vi "Begin.vi"() -> (0 "error out":errorcluster)   [LabVIEW 2013]
doc: "Called before other user functions, this VI is expected to open initial I/O refnums, load in file data, and do all program initialization. Notice that the <B>error out</B> terminal is simply used for data flow. Wiring it to other structures or subVIs ensures that this VI runs first."
uses:
  <vilib>/Rock Robotics/SystemInterfaces/DIO/FPGA_DIOPWMChannel.ctl
  <vilib>/Rock Robotics/WPI/DriverStation/WPI_DriverStationRobotMode2.ctl
  <vilib>/Rock Robotics/WPI/Joystick/WPI_JoystickDeviceEnum.ctl
  <vilib>/Rock Robotics/WPI/Solenoid/WPI_SolenoidChannel.ctl
  <vilib>/Rock Robotics/SystemInterfaces/DIO/FPGA_DIOChannel.ctl
  <vilib>/Rock Robotics/SystemInterfaces/DIO/FPGA_DIORelayChannel.ctl
  <vilib>/Rock Robotics/SystemInterfaces/Typedef/FPGA_TypedefAnalogModule.ctl
  <vilib>/Rock Robotics/SystemInterfaces/AI/FPGA_AIChannel.ctl
  <vilib>/Rock Robotics/WPI/RobotDrive/WPI_RobotDriveOpen2MotorWithTalon.vi
  Robot Global Data.vi
  <vilib>/Rock Robotics/WPI/MotorControl/WPI_MotorControlOpen Jaguar.vi
  <vilib>/Rock Robotics/WPI/Solenoid/WPI_SolenoidOpenDouble.vi
  <vilib>/Rock Robotics/WPI/Compressor/WPI_CompressorGetSetRefNum.vi
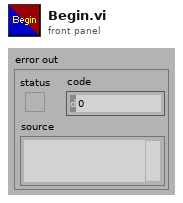
[diagram p1: front panel]
types:
  T1 = typedef "FPGA_AIChannel.ctl" = enum8{"AI 1", "AI 2", "AI 3", "AI 4", "AI 5", "AI 6", "AI 7", "AI 8", "Invalid"}
  T2 = typedef "FPGA_TypedefAnalogModule.ctl" = enum16{"Analog Module 1", "Analog Module 2"}
  T3 = typedef "FPGA_DIOChannel.ctl" = enum8{"DIO 1", "DIO 2", "DIO 3", "DIO 4", "DIO 5", "DIO 6", "DIO 7", "DIO 8", "DIO 9", "DIO 10", "DIO 11", "DIO 12", "DIO 13", "DIO 14", "Invalid"}
  T4 = typedef "WPI_SolenoidChannel.ctl" = enum8{"Solenoid 1", "Solenoid 2", "Solenoid 3", "Solenoid 4", "Solenoid 5", "Solenoid 6", "Solenoid 7", "Solenoid 8", "Invalid"}
  T5 = typedef "FPGA_DIORelayChannel.ctl" = enum8{"Relay 1", "Relay 2", "Relay 3", "Relay 4", "Relay 5", "Relay 6", "Relay 7", "Relay 8", "Invalid"}
  T6 = typedef "FPGA_DIOPWMChannel.ctl" = enum8{"PWM 1", "PWM 2", "PWM 3", "PWM 4", "PWM 5", "PWM 6", "PWM 7", "PWM 8", "PWM 9", "PWM 10", "Invalid"}
  T7 = typedef "WPI_JoystickDeviceEnum.ctl" = enum16{"USB 1", "USB 2", "USB 3", "USB 4", "Kinect 1", "Kinect 2"}
  T8 = typedef "WPI_DriverStationRobotMode2.ctl" = enum16{"Autonomous Disabled", "Autonomous Enabled", "Teleop Disabled", "Teleop Enabled", "Timeout", "Finish", "Test Disabled", "Test Enabled"}
  T9 = typedef "WPI_AnalogChannelDevRef.ctl" = cluster{"DevStatus":errorcluster, "Analog Module":T2, "Analog Channel":T1}
  T10 = typedef "WPI_DigitalInputDevRef.ctl" = cluster{"DevStatus":errorcluster, "DIO Channel":T3, "Digital Module":T11}
  T11 = typedef "FPGA_TypedefDigitalModule.ctl" = enum16{"Digital Module 1", "Digital Module 2"}
  T12 = typedef "WPI_MotorControlDeviceRef.ctl" = cluster{"DeviceStatus":errorcluster, "Type":enum16{"PWM", "CAN"}, "PWM":cluster{"Digital Module":T11, "PWM Channel":T6, "DeadBand":T13}, "CAN":cluster{"Device Number":u8, "Control Mode":T14, "Semaphore":T15, "Max Vout":dbl}, "Invert":bool, "TransformRef":T16, "InvTransformRef":T16}
  T13 = typedef "WPI_PWMDeadband.ctl" = cluster{"Name":string, "maxPositivePwm":i32, "minPositivePwm":i32, "centerPwm":i32, "maxNegativePwm":i32, "minNegativePwm":i32, "angularRange":u16}
  T14 = typedef "WPI_CANJaguar_ControlMode.ctl" = enum8{"Percent VBus", "Current", "Speed", "Position", "Voltage"}
  T15 = typedef "Semaphore RefNum" = refnum<k1>
  T16 = typedef "WPI_PWMTransform_ConPane.ctl" = refnum<vi>
  T17 = typedef "WPI_ServoDeviceRef.ctl" = cluster{"DeviceStatus":errorcluster, "Digital Module":T11, "PWM Channel":T6, "DeadBand":T13}
  T18 = typedef "WPI_RobotDriveDevRef.ctl" = cluster{"DevStatus":errorcluster, "Motors[]":T12[], "Square Inputs":bool, "Max Output":dbl, "Isochronous":bool}
  T19 = typedef "WPI_JoystickDevRef.ctl" = cluster{"Device":T7}
  T20 = typedef "WPI_RelayDevRef.ctl" = cluster{"DevStatus":errorcluster, "Relay Channel":T5, "Digital Module":T11, "Relay Direction":T21}
  T21 = typedef "WPI_RelayDirection.ctl" = enum16{"Both directions", "Forward only", "Reverse only"}
  T22 = typedef "WPI_CompressorDevRef.ctl" = cluster{"DevStatus":errorcluster, "DigitalInputDevRef":T10, "RelayDevRef":T20}
  T23 = typedef "WPI_SolenoidDevRef.ctl" = cluster{"DevStatus":errorcluster, "Solenoid Module":T24, "Forward Solenoid Channel":T4, "Reverse Solenoid Channel":T4}
  T24 = typedef "FPGA_TypedefSolenoidModule.ctl" = enum16{"Solenoid Module 1", "Solenoid Module 2"}
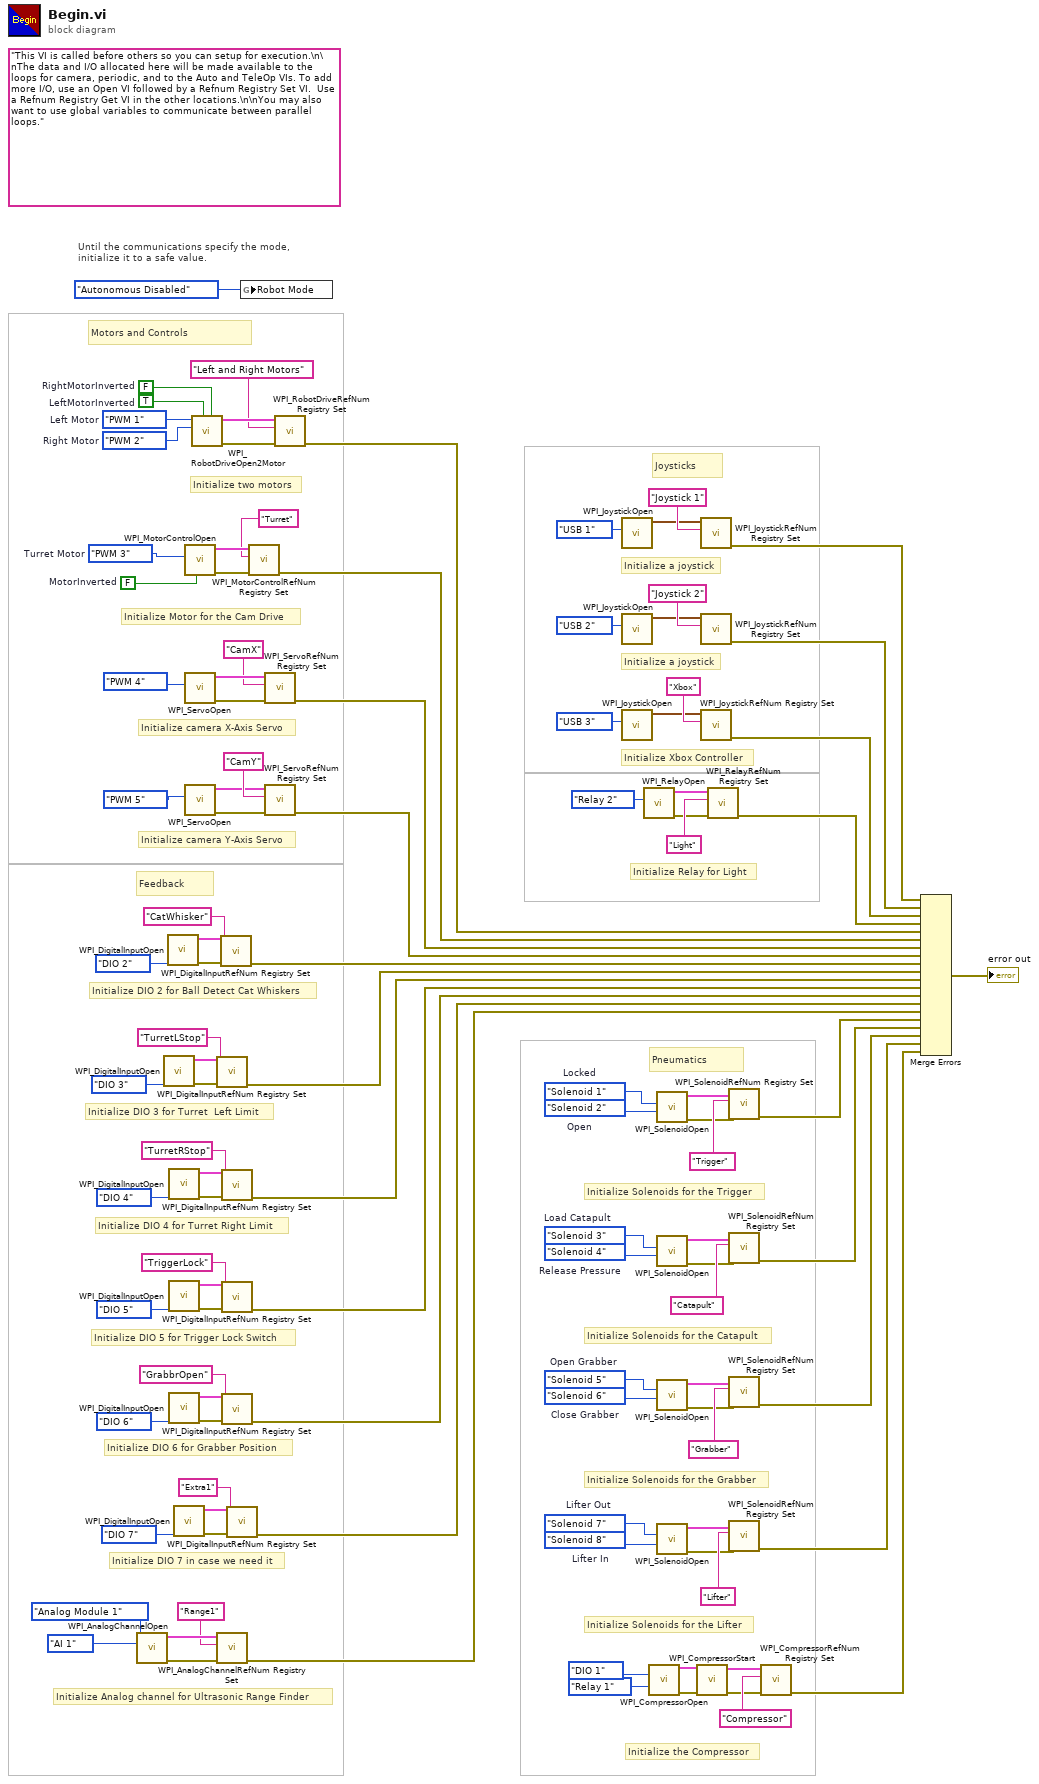
[diagram p0: block diagram]
diagram:
  w32 = WPI_SolenoidChannel."Solenoid 8"  # Lifter In
  w33 = WPI_SolenoidChannel."Solenoid 6"  # Close Grabber
  w34 = WPI_SolenoidChannel."Solenoid 4"  # Release Pressure
  w35 = WPI_SolenoidChannel."Solenoid 2"  # Open
  w51 = FALSE  # MotorInverted
  w55 = FPGA_DIOPWMChannel."PWM 3"  # Turret Motor
  w83 = WPI_SolenoidChannel."Solenoid 7"  # Lifter Out
  w86 = WPI_SolenoidChannel."Solenoid 5"  # Open Grabber
  w89 = WPI_SolenoidChannel."Solenoid 3"  # Load Catapult
  w92 = WPI_SolenoidChannel."Solenoid 1"  # Locked
  (unwired) "This VI is called before others so you can setup for execution.\n\nThe data and I/O allocated here will be made available to the loops for camera, periodic, and to the Auto and TeleOp VIs. To add more I/O, use an Open VI followed by a Refnum Registry Set VI.  Use a Refnum Registry Get VI in the other locations.\n\nYou may also want to use global variables to communicate between parallel loops."
  w105 = FPGA_DIOPWMChannel."PWM 2"  # Right Motor
  w106 = FPGA_DIOPWMChannel."PWM 1"  # Left Motor
  w110 = TRUE  # LeftMotorInverted
  w111 = FALSE  # RightMotorInverted
  # "Initialize DIO 2 for Ball Detect Cat Whiskers"
  # "Initialize the Compressor"
  # "Joysticks"
  # "Initialize DIO 7 in case we need it"
  # "Initialize DIO 3 for Turret  Left Limit"
  # "Initialize DIO 6 for Grabber Position"
  # "Initialize DIO 5 for Trigger Lock Switch"
  # "Initialize DIO 4 for Turret Right Limit"
  # "Initialize Analog channel for Ultrasonic Range Finder"
  # "Initialize camera Y-Axis Servo"
  # "Initialize camera X-Axis Servo"
  # "Initialize Relay for Light"
  # "Initialize Motor for the Cam Drive"
  # "Initialize Solenoids for the Lifter"
  # "Initialize Solenoids for the Grabber"
  # "Initialize Solenoids for the Catapult"
  # "Initialize Solenoids for the Trigger"
  # "Feedback"
  # "Pneumatics"
  # "Motors and Controls"
  # "Initialize Xbox Controller"
  # "Initialize a joystick"
  # "Initialize a joystick"
  # "Until the communications specify the mode,\ninitialize it to a safe value."
  # "Initialize two motors"
  n1 = call <vilib>:"WPI_AnalogChannelOpen.vi"("Analog Channel"=FPGA_AIChannel."AI 1", "Analog Module (Module 1)"=FPGA_TypedefAnalogModule."Analog Module 1") -> ("error out"=w11:errorcluster, "AIDeviceRef"=w10:T9)  [unwired: 8 in]
  n2 = call <vilib>:"WPI_DigitalInputOpen.vi"("DIO Channel"=FPGA_DIOChannel."DIO 3") -> ("error out"=w13:errorcluster, "DigitalInputDevRef"=w73:T10)  [unwired: 9 in]
  n3 = call <vilib>:"WPI_DigitalInputOpen.vi"("DIO Channel"=FPGA_DIOChannel."DIO 2") -> ("error out"=w12:errorcluster, "DigitalInputDevRef"=w31:T10)  [unwired: 9 in]
  n4 = call <vilib>:"WPI_DigitalInputOpen.vi"("DIO Channel"=FPGA_DIOChannel."DIO 4") -> ("error out"=w14:errorcluster, "DigitalInputDevRef"=w82:T10)  [unwired: 9 in]
  n5 = call <vilib>:"WPI_DigitalInputOpen.vi"("DIO Channel"=FPGA_DIOChannel."DIO 5") -> ("error out"=w15:errorcluster, "DigitalInputDevRef"=w79:T10)  [unwired: 9 in]
  n6 = call <vilib>:"WPI_DigitalInputOpen.vi"("DIO Channel"=FPGA_DIOChannel."DIO 6") -> ("error out"=w16:errorcluster, "DigitalInputDevRef"=w76:T10)  [unwired: 9 in]
  n7 = call <vilib>:"WPI_DigitalInputOpen.vi"("DIO Channel"=FPGA_DIOChannel."DIO 7") -> ("error out"=w17:errorcluster, "DigitalInputDevRef"=w70:T10)  [unwired: 9 in]
  n8 = call-poly <vilib>:"WPI_MotorControlOpen.vi"("Invert"=w51, "PWM Channel"=w55) -> ("error out"=w53:errorcluster, "MotorControlDeviceRef"=w54:T12)  [unwired: 8 in]
  n9 = call <vilib>:"WPI_ServoOpen.vi"("PWM Channel"=FPGA_DIOPWMChannel."PWM 4" ("X Channel")) -> ("error out"=w61:errorcluster, "ServoDeviceRef"=w60:T17)  [unwired: 3 in, 6 out]
  n10 = call <vilib>:"WPI_ServoOpen.vi"("PWM Channel"=FPGA_DIOPWMChannel."PWM 5" ("Y Channel")) -> ("error out"=w56:errorcluster, "ServoDeviceRef"=w57:T17)  [unwired: 3 in, 6 out]
  n11 = call-poly <vilib>:"WPI_RobotDriveOpen2Motor.vi"("Right Motor Inverted"=w111, "Left Motor Inverted"=w110, "Right Motor"=w105, "Left Motor"=w106) -> ("error out"=w107:errorcluster, "RobotDriveDevRef"=w109:T18)  [unwired: 1 in, 5 out]
  n12 = call <vilib>:"WPI_DigitalInputRefNum Registry Set.vi"("error in (no error)"=w13, "refnum name"="TurretLStop", "DigitalInputDevRef"=w73) -> ("error out"=w46:errorcluster)  [unwired: 7 in, 1 out]
  n13 = call <vilib>:"WPI_AnalogChannelRefNum Registry Set.vi"("error in (no error)"=w11, "refnum name"="Range1", "AIDeviceRef"=w10) -> ("error out"=w6:errorcluster)  [unwired: 7 in, 1 out]
  n14 = call <vilib>:"WPI_DigitalInputRefNum Registry Set.vi"("error in (no error)"=w12, "refnum name"="CatWhisker", "DigitalInputDevRef"=w31) -> ("error out"=w28:errorcluster)  [unwired: 7 in, 1 out]
  n15 = call <vilib>:"WPI_DigitalInputRefNum Registry Set.vi"("error in (no error)"=w14, "refnum name"="TurretRStop", "DigitalInputDevRef"=w82) -> ("error out"=w45:errorcluster)  [unwired: 7 in, 1 out]
  n16 = call <vilib>:"WPI_DigitalInputRefNum Registry Set.vi"("error in (no error)"=w15, "refnum name"="TriggerLock", "DigitalInputDevRef"=w79) -> ("error out"=w44:errorcluster)  [unwired: 7 in, 1 out]
  n17 = call <vilib>:"WPI_DigitalInputRefNum Registry Set.vi"("error in (no error)"=w16, "refnum name"="GrabbrOpen", "DigitalInputDevRef"=w76) -> ("error out"=w43:errorcluster)  [unwired: 7 in, 1 out]
  n18 = call <vilib>:"WPI_DigitalInputRefNum Registry Set.vi"("error in (no error)"=w17, "refnum name"="Extra1", "DigitalInputDevRef"=w70) -> ("error out"=w42:errorcluster)  [unwired: 7 in, 1 out]
  n19 = global write "Robot Global Data.vi" "Robot Mode"(WPI_DriverStationRobotMode2."Autonomous Disabled" ("Robot Mode")) -> ()
  n20 = call <vilib>:"WPI_MotorControlRefNum Registry Set.vi"("error in (no error)"=w53, "refnum name"="Turret", "MotorControlDevRef"=w54) -> ("error out"=w49:errorcluster)  [unwired: 7 in, 1 out]
  n21 = call <vilib>:"WPI_ServoRefNum Registry Set.vi"("error in (no error)"=w61, "refnum name"="CamX", "ServoDeviceRef"=w60) -> ("error out"=w48:errorcluster)  [unwired: 7 in, 1 out]
  n22 = call <vilib>:"WPI_ServoRefNum Registry Set.vi"("error in (no error)"=w56, "refnum name"="CamY", "ServoDeviceRef"=w57) -> ("error out"=w47:errorcluster)  [unwired: 7 in, 1 out]
  n23 = call <vilib>:"WPI_RobotDriveRefNum Registry Set.vi"("error in (no error)"=w107, "refnum name"="Left and Right Motors", "RobotDriveDevRef"=w109) -> ("error out"=w50:errorcluster)  [unwired: 8 out]
  n24 = call <vilib>:"WPI_JoystickOpen.vi"("JoystickDevice"=WPI_JoystickDeviceEnum."USB 1") -> ("JoystickDevRef"=w102:T19)  [unwired: 10 in]
  n25 = call <vilib>:"WPI_JoystickOpen.vi"("JoystickDevice"=WPI_JoystickDeviceEnum."USB 2") -> ("JoystickDevRef"=w99:T19)  [unwired: 10 in]
  n26 = call <vilib>:"WPI_JoystickOpen.vi"("JoystickDevice"=WPI_JoystickDeviceEnum."USB 3") -> ("JoystickDevRef"=w96:T19)  [unwired: 10 in]
  n27 = call <vilib>:"WPI_RelayOpen.vi"("Relay Channel"=FPGA_DIORelayChannel."Relay 2") -> ("error out"=w65:errorcluster, "RelayDevRef"=w66:T20)  [unwired: 9 in]
  n28 = call <vilib>:"WPI_CompressorOpen.vi"("Pressure Switch DIO Channel"=FPGA_DIOChannel."DIO 1", "Relay Channel"=FPGA_DIORelayChannel."Relay 1") -> ("CompressorDevRef"=w36:T22, "error out"=w23:errorcluster)  [unwired: 12 in]
  n29 = call-poly <vilib>:"WPI_SolenoidOpen.vi"("Reverse Solenoid Channel"=w35, "Forward Solenoid Channel"=w92) -> ("error out"=w18:errorcluster, "SolenoidDevRef"=w94:T23)  [unwired: 8 in]
  n30 = call-poly <vilib>:"WPI_SolenoidOpen.vi"("Reverse Solenoid Channel"=w34, "Forward Solenoid Channel"=w89) -> ("error out"=w19:errorcluster, "SolenoidDevRef"=w91:T23)  [unwired: 8 in]
  n31 = call-poly <vilib>:"WPI_SolenoidOpen.vi"("Reverse Solenoid Channel"=w33, "Forward Solenoid Channel"=w86) -> ("error out"=w20:errorcluster, "SolenoidDevRef"=w88:T23)  [unwired: 8 in]
  n32 = call-poly <vilib>:"WPI_SolenoidOpen.vi"("Reverse Solenoid Channel"=w32, "Forward Solenoid Channel"=w83) -> ("error out"=w21:errorcluster, "SolenoidDevRef"=w85:T23)  [unwired: 8 in]
  n33 = call <vilib>:"WPI_CompressorStart.vi"("error in (no error)"=w23, "CompressorDevRef"=w36) -> ("error out"=w22:errorcluster, "CompressorDevRef"=w40:T22)  [unwired: 8 in]
  n34 = call <vilib>:"WPI_JoystickRefNum Registry Set.vi"("refnum name"="Joystick 1", "JoystickDevRef"=w102) -> ("error out"=w24:errorcluster)  [unwired: 8 in, 1 out]
  n35 = call <vilib>:"WPI_JoystickRefNum Registry Set.vi"("refnum name"="Joystick 2", "JoystickDevRef"=w99) -> ("error out"=w25:errorcluster)  [unwired: 8 in, 1 out]
  n36 = call <vilib>:"WPI_JoystickRefNum Registry Set.vi"("refnum name"="Xbox", "JoystickDevRef"=w96) -> ("error out"=w26:errorcluster)  [unwired: 8 in, 1 out]
  n37 = call <vilib>:"WPI_RelayRefNum Registry Set.vi"("error in (no error)"=w65, "refnum name"="Light", "RelayDevRef"=w66) -> ("error out"=w27:errorcluster)  [unwired: 7 in, 1 out]
  n38 = call <vilib>:"WPI_SolenoidRefNum Registry Set.vi"("error in (no error)"=w18, "refnum name"="Trigger", "SolenoidDevRef"=w94) -> ("error out"=w5:errorcluster)  [unwired: 7 in, 1 out]
  n39 = call <vilib>:"WPI_SolenoidRefNum Registry Set.vi"("error in (no error)"=w19, "refnum name"="Catapult", "SolenoidDevRef"=w91) -> ("error out"=w4:errorcluster)  [unwired: 7 in, 1 out]
  n40 = call <vilib>:"WPI_SolenoidRefNum Registry Set.vi"("error in (no error)"=w20, "refnum name"="Grabber", "SolenoidDevRef"=w88) -> ("error out"=w3:errorcluster)  [unwired: 7 in, 1 out]
  n41 = call <vilib>:"WPI_SolenoidRefNum Registry Set.vi"("error in (no error)"=w21, "refnum name"="Lifter", "SolenoidDevRef"=w85) -> ("error out"=w2:errorcluster)  [unwired: 7 in, 1 out]
  n42 = call <vilib>:"WPI_CompressorRefNum Registry Set.vi"("error in (no error)"=w22, "refnum name"="Compressor", "CompressorDevRef"=w40) -> ("error out"=w1:errorcluster)  [unwired: 7 in, 1 out]
  n43 = Merge Errors(w24, w25, w26, w27, w50, w49, w48, w47, w28, w46, w45, w44, w43, w42, w6, w5, w4, w3, w2, w1) -> (→"error out":errorcluster)
